vi "Batch Linear Regression.vi"() -> ()   [LabVIEW 2020]
panel:
  out "error out":errorcluster
  out "?":string[][](table)
  out "Origin ogw Load":bool
  out "ogw path":path
  in  "Visible":i32(ring) caption="Origin Visible" items=["MAINWND_HIDE"=0, "MAINWND_SHOW"=1, "MAINWND_SHOWMINIMIZED"=2, "MAINWND_SHOWMAXIMIZED"=3, "MAINWND_SHOW_BRING_TO_FRONT"=100]
  # "Please note that a dialog will be prompted to ask you to select one or multiple data files. To be compatible with the customized analysis template, you should select the \"Sensor01.dat\", \"Sensor02.dat\" and \"Sensor03.dat\" together (or just select one of them) that in the <Origin Program Folder>\\Samples\\Curve Fitting folder.\n\nThis VI mainly shows you to do the following two things:\n\n1. Get and change existing Linear Fit operation that stored in the Analysis Template. \n2. Perform Batch Processing with the modified analysis template and then return the results."
  # "Note: \n\n1. Get and change existing Linear Fit operation that stored in the Analysis Template. \n2. Perform Batch Processing with the modified analysis template and then returen the results."
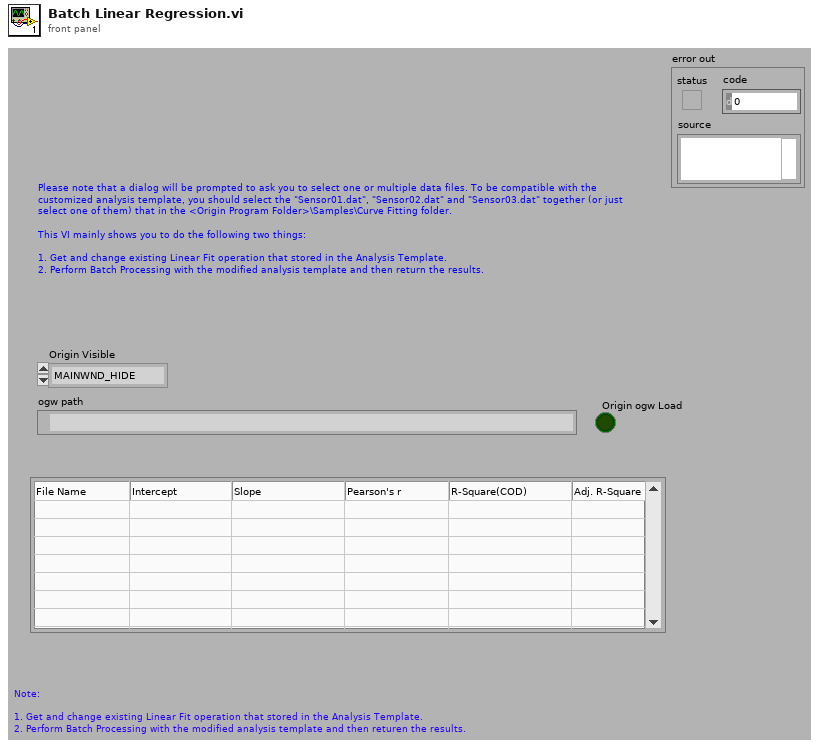
[diagram p1: front panel]
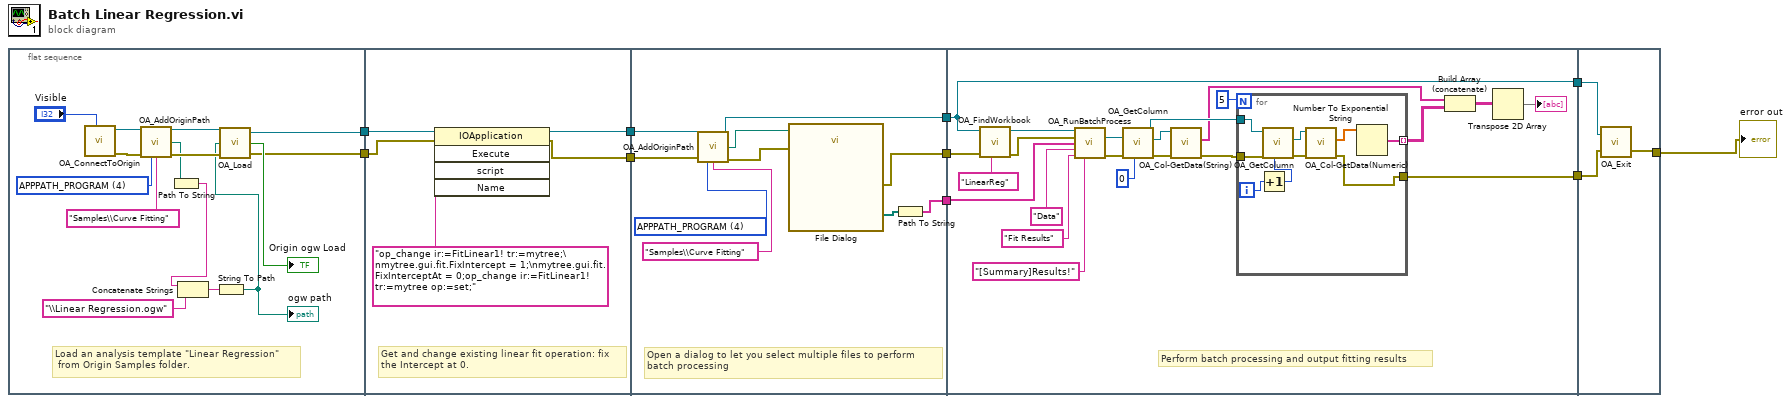
[diagram p0: block diagram]
diagram:
  n1 = flat-sequence {
    tunnel: [w12] -> w8
    tunnel: [w11] -> w7
    tunnel: w8 -> [w30]
    tunnel: w7 -> [w29]
    tunnel: [w27] -> w6
    tunnel: [w26] -> w5
    tunnel: [w36] -> w10
    tunnel: [w34] -> w9
    tunnel: w6 -> [w33]
    tunnel: w5 -> [w32]
    tunnel: [w31] -> w4
    tunnel: w10 -> [w42]
    tunnel: w9 -> [w46]
    tunnel: w4 -> [w44]
    tunnel: [w45] -> w3
    tunnel: [w44] -> w2
    tunnel: w3 -> [w73]
    tunnel: w2 -> [w74]
    tunnel: [w72] -> w1
    frame #0 {
      w23 = 4 items=["APPPATH_USER"=2, "APPPATH_GROUP"=3, "APPPATH_PROGRAM"=4] ("Type")
      # "Load an analysis template \"Linear Regression\" \n from Origin Samples folder."
      n2 = call "OA_ConnectToOrigin.vi"("Visible"="Visible") -> ("error out"=w20:errorcluster, "Origin.IOApplication"=w21:refnum<k7>)  [unwired: 7 in]
      n3 = call "OA_AddOriginPath.vi"("Origin.IOApplication"=w21, "error in (no error)"=w20, "Type"=w23, "Filename"="Samples\\Curve Fitting") -> ("Origin.IOApplication"=w25:refnum<k7>, "path out"=w15:path, "error out"=w24:errorcluster)  [unwired: 9 in]
      n4 = Path To String(path=w15) -> (string=w13:string)
      n5 = Concatenate Strings(w13, "\\Linear Regression.ogw" ("string")) -> (w17:string)
      n6 = String To Path(string=w17) -> (path=w16:path)
      "ogw path" <- w16
      n7 = call "OA_Load.vi"("error in (no error)"=w24, "Path"=w16, "Origin.IOApplication"=w25) -> ("error out"=w11:errorcluster, "Load"=→"Origin ogw Load":bool, "Origin.IOApplication"=w12:refnum<k7>)
    }
    frame #1 {
      # "Get and change existing linear fit operation: fix\nthe Intercept at 0."
      n8 = invoke class="IOApplication" method="Execute"(reference=w30, error in=w29, "script"="op_change ir:=FitLinear1! tr:=mytree;\nmytree.gui.fit.FixIntercept = 1;\nmytree.gui.fit.FixInterceptAt = 0;op_change ir:=FitLinear1! tr:=mytree op:=set;" ("LabTalkStr")) -> (reference out=w27:refnum<k7>, error out=w26:errorcluster)  [unwired: 2 in, 3 out]
    }
    frame #2 {
      w40 = 4 items=["APPPATH_USER"=2, "APPPATH_GROUP"=3, "APPPATH_PROGRAM"=4] ("Type")
      # "Open a dialog to let you select multiple files to perform \nbatch processing"
      n9 = call "OA_AddOriginPath.vi"("Origin.IOApplication"=w33, "error in (no error)"=w32, "Type"=w40, "Filename"="Samples\\Curve Fitting") -> ("Origin.IOApplication"=w31:refnum<k7>, "path out"=w38:path, "error out"=w37:errorcluster)  [unwired: 9 in]
      n10 = call "File Dialog"("start path"=w38, "error in"=w37) -> ("selected paths"=w35:path[], "error out"=w36:errorcluster)  [unwired: 10 in, 2 out]
      n11 = Path To String(path=w35) -> (string=w34:string[])
    }
    frame #3 {
      # "Perform batch processing and output fitting results"
      n12 = call "OA_FindWorkbook.vi"("Book Name"="LinearReg", "error in (no error)"=w42, "Origin.IOApplication"=w44) -> ("error out"=w58:errorcluster, "Origin.WorksheetPage Out"=w59:refnum<k7>)  [unwired: 7 in]
      n13 = call "OA_RunBatchProcess.vi"("Origin.WorksheetPage"=w59, "error in (no error)"=w58, "File List"=w46, "Data Sheet"="Data" ("Data Sheet Name"), "Result Sheet"="Fit Results" ("Result Sheet Name"), "Output Sheet"="[Summary]Results!") -> ("Origin.Output Worksheet"=w55:refnum<k7>, "error out"=w54:errorcluster)  [unwired: 7 in, 1 out]
      n14 = call "OA_GetColumn.vi"("Column Name/Index"=0, "error in (no error)"=w54, "Origin.Worksheet"=w55) -> ("error out"=w62:errorcluster, "Origin.Column"=w61:refnum<k7>, "Origin.Worksheet"=w51:refnum<k7>)  [unwired: 6 in]
      n15 = call "OA_Col-GetData(String).vi"("error in (no error)"=w62, "Origin.Column"=w61) -> ("error out"=w41:errorcluster, "data"=w49:string[])  [unwired: 7 in, 1 out]
      n16 = for {
        N: 5 -> [_]
        tunnel: w41 -> [w69]
        tunnel: w51 -> [w65]
        tunnel: [w63] -> w45
        tunnel: [w64] -> w50 mode=indexing
        i -> [w71]
        n17 = Increment(x=w71) -> (x+1=w70:i32)
        n18 = call "OA_GetColumn.vi"("Column Name/Index"=w70, "error in (no error)"=w69, "Origin.Worksheet"=w65) -> ("error out"=w68:errorcluster, "Origin.Column"=w67:refnum<k7>)  [unwired: 6 in, 1 out]
        n19 = call "OA_Col-GetData(Numeric).vi"("error in (no error)"=w68, "Origin.Column"=w67) -> ("error out"=w63:errorcluster, "data"=w66:dbl[])  [unwired: 7 in, 1 out]
        n20 = Number To Exponential String(number=w66) -> (E-format string=w64:string[])  [unwired: 3 in]
      }
      n21 = Build Array (concatenate)(w49, w50) -> (w48:string[][])
      n22 = Transpose 2D Array(2D array=w48) -> (transposed array=→"?":string[][])
    }
    frame #4 {
      n23 = call "OA_Exit.vi"("Error IO"=w73, "Origin.IOApplication"=w74) -> ("Error IO Out"=w72:errorcluster)  [unwired: 1 out]
    }
  }
  "error out" <- w1
